vi "Periodic Tasks.vi"(8 "error in":errorcluster) -> ()   [LabVIEW 2013]
doc: "This VI runs in parallel to other tasks. It can contain as many user-defined periodic loops as you need. These can carry out PID or other sorts of timed response."
uses:
  <vilib>/Rock Robotics/SystemInterfaces/Utilities/FPGA_UtilitiesLED Source.ctl
  <vilib>/Rock Robotics/SystemInterfaces/Utilities/FPGA_UtilitiesLED State.ctl
  Robot Global Data.vi
panel:
  out "RDistance":dbl
  out "LDistance":dbl
  out "Distance":dbl
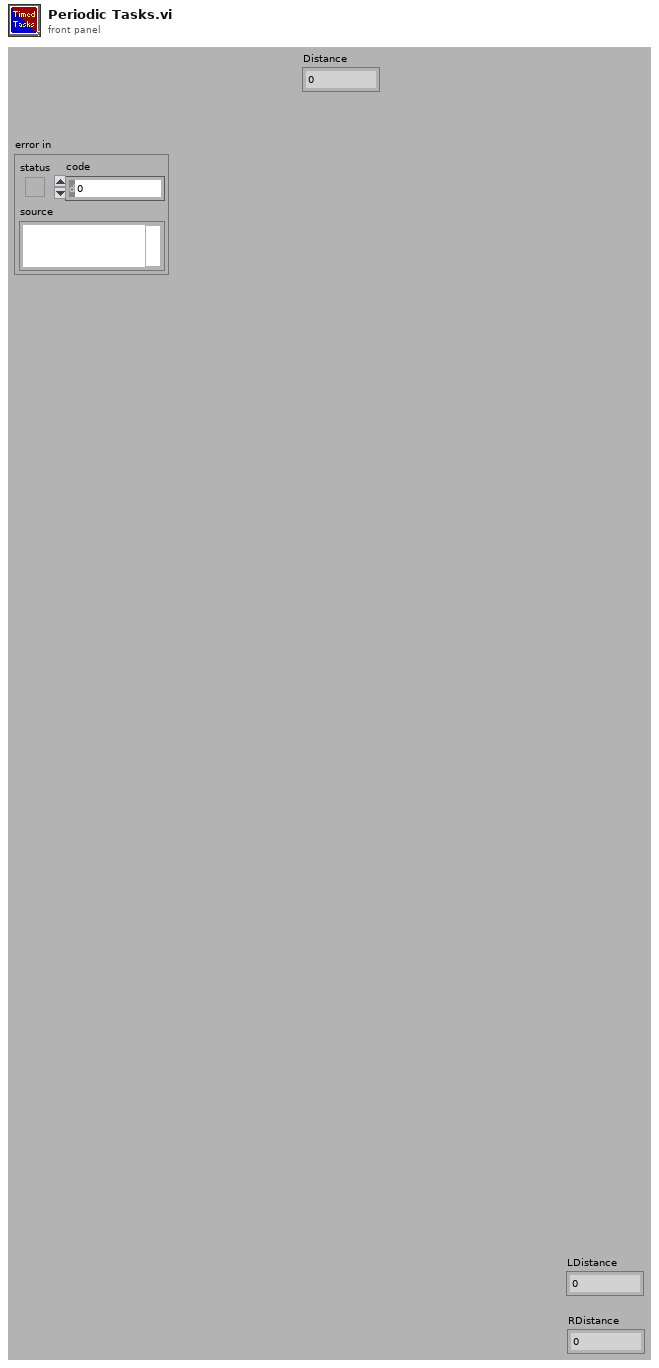
[diagram p1: front panel]
types:
  T1 = typedef "WPI_AnalogChannelDevRef.ctl" = cluster{"DevStatus":errorcluster, "Analog Module":T2, "Analog Channel":T3}
  T2 = typedef "FPGA_TypedefAnalogModule.ctl" = enum16{"Analog Module 1", "Analog Module 2"}
  T3 = typedef "FPGA_AIChannel.ctl" = enum8{"AI 1", "AI 2", "AI 3", "AI 4", "AI 5", "AI 6", "AI 7", "AI 8", "Invalid"}
  T4 = typedef "WPI_DigitalInputDevRef.ctl" = cluster{"DevStatus":errorcluster, "DIO Channel":T5, "Digital Module":T6}
  T5 = typedef "FPGA_DIOChannel.ctl" = enum8{"DIO 1", "DIO 2", "DIO 3", "DIO 4", "DIO 5", "DIO 6", "DIO 7", "DIO 8", "DIO 9", "DIO 10", "DIO 11", "DIO 12", "DIO 13", "DIO 14", "Invalid"}
  T6 = typedef "FPGA_TypedefDigitalModule.ctl" = enum16{"Digital Module 1", "Digital Module 2"}
  T7 = typedef "WPI_EncoderDevRef.ctl" = cluster{"DevStatus":errorcluster, "EncoderIndex":T8, "CounterIndex":T9, "DistancePerCount":dbl, "Decoding Type":T10}
  T8 = typedef "FPGA_EncoderIdx.ctl" = enum8{"Enc 0", "Enc 1", "Enc 2", "Enc 3", "Invalid"}
  T9 = typedef "FPGA_CounterCtrSystemIndex.ctl" = enum8{"Ctr 0", "Ctr 1", "Ctr 2", "Ctr 3", "Ctr 4", "Ctr 5", "Ctr 6", "Ctr 7", "Invalid"}
  T10 = typedef "WPI_EncoderType.ctl" = enum16{"1x", "2x", "4x"}
  T11 = cluster{"Winch Desired Location":dbl, "Winch Desired Location 2":dbl, "Winch Desired Location 3":dbl}
  T12 = typedef "FPGA_UtilitiesLED State.ctl" = enum16{"Off", "On", "Toggle"}
  T13 = typedef "FPGA_UtilitiesLED Source.ctl" = enum16{"User LED", "FPGA LED"}
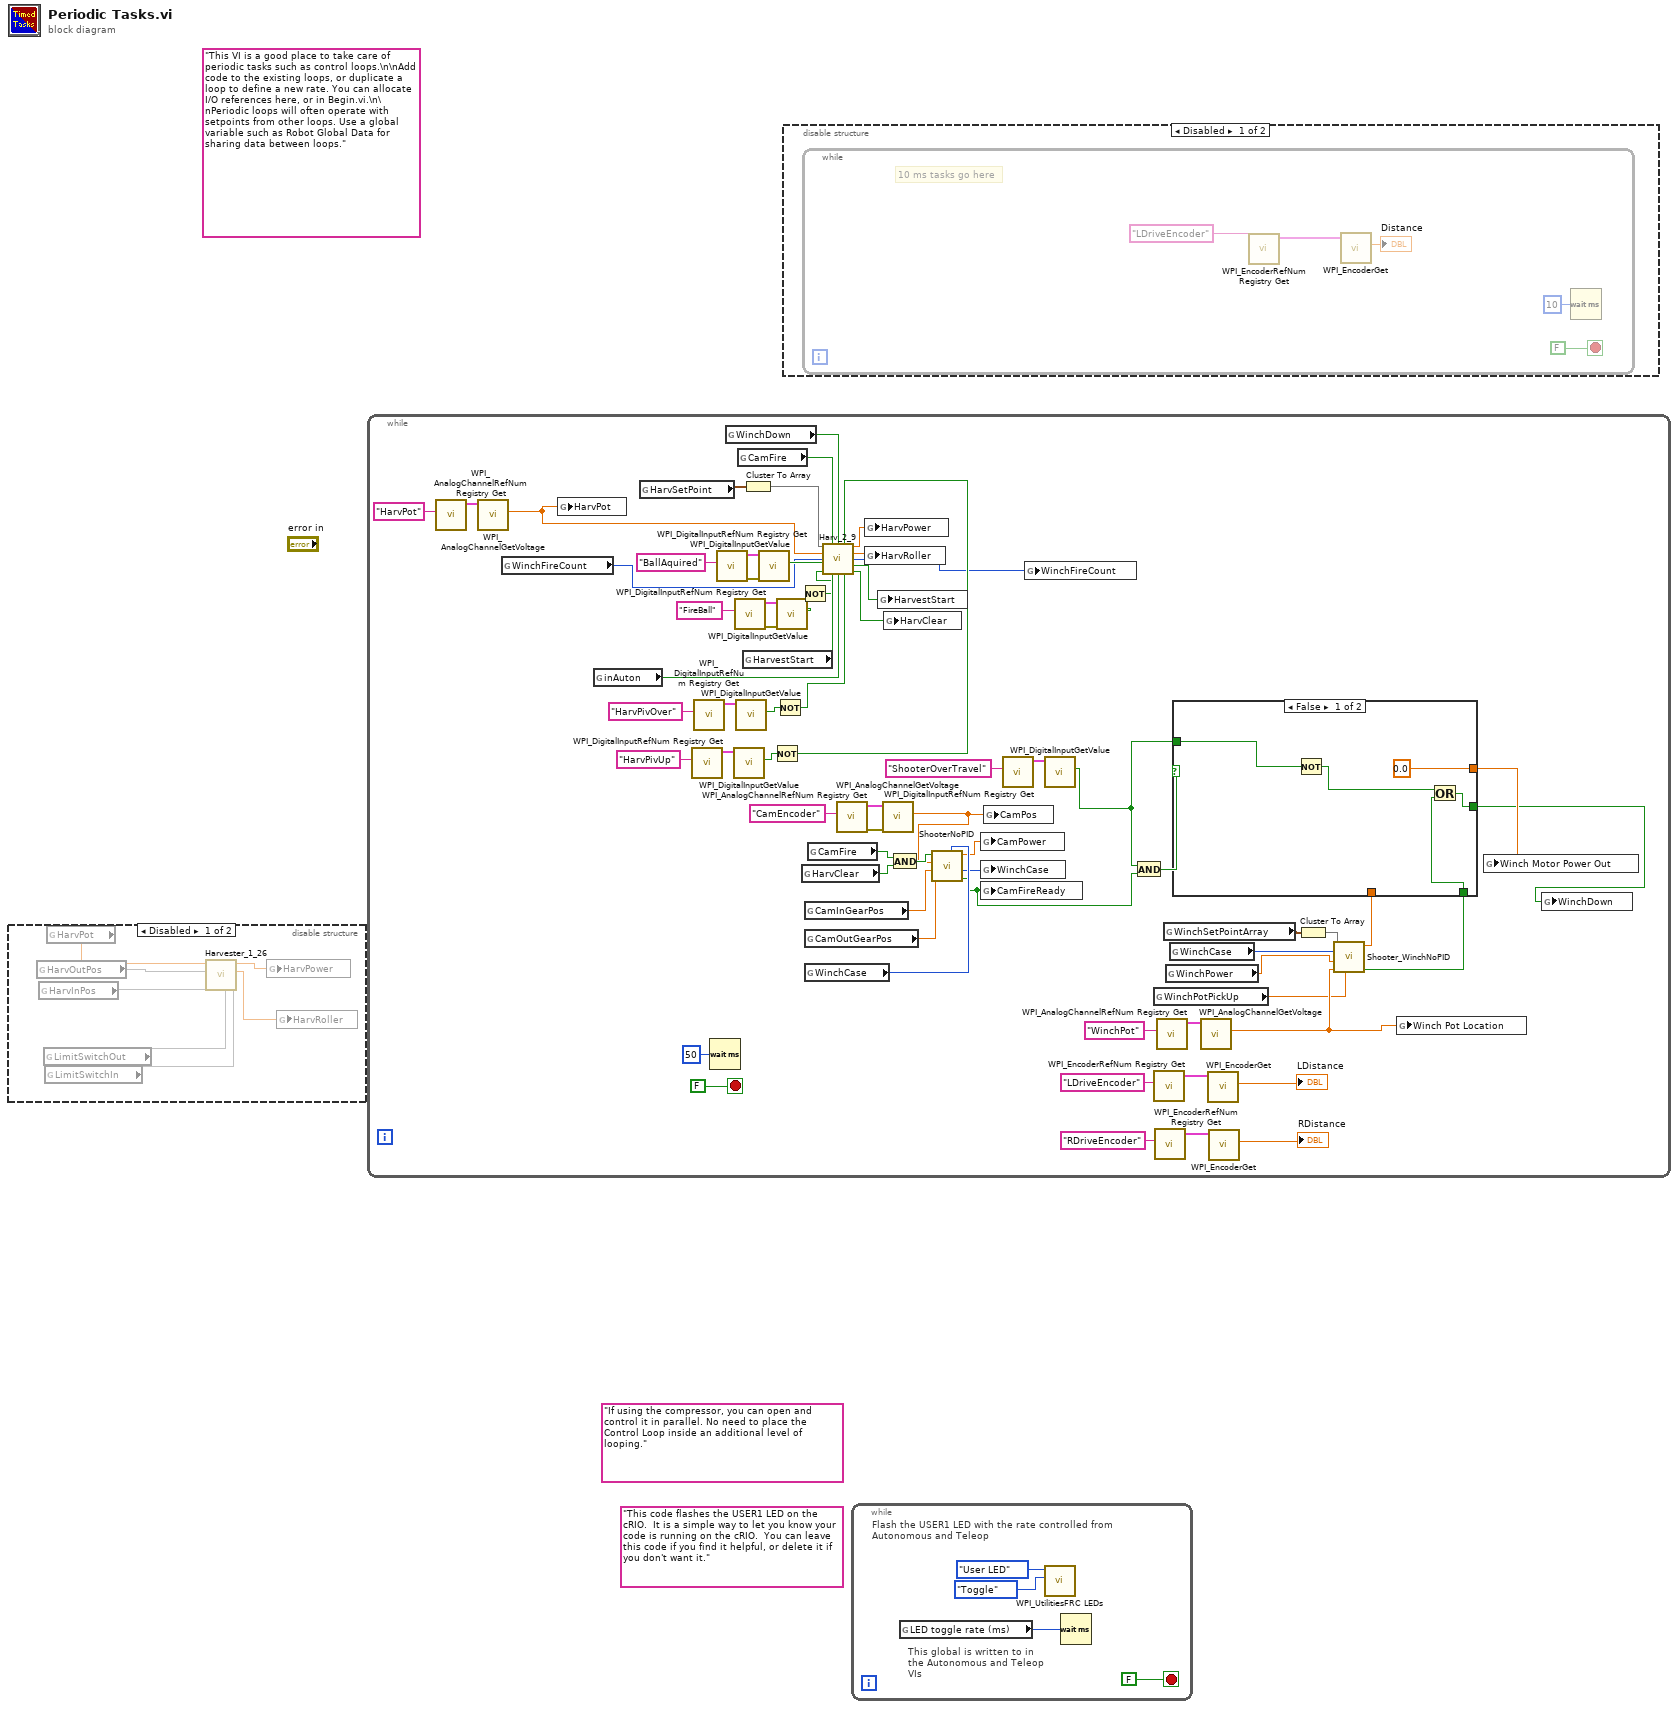
[diagram p0: block diagram]
diagram:
  (unwired) "If using the compressor, you can open and control it in parallel. No need to place the Control Loop inside an additional level of looping."
  (unwired) "This code flashes the USER1 LED on the cRIO.  It is a simple way to let you know your code is running on the cRIO.  You can leave this code if you find it helpful, or delete it if you don't want it."
  (unwired) "This VI is a good place to take care of periodic tasks such as control loops.\n\nAdd code to the existing loops, or duplicate a loop to define a new rate. You can allocate I/O references here, or in Begin.vi.\n\nPeriodic loops will often operate with setpoints from other loops. Use a global variable such as Robot Global Data for sharing data between loops."
  n1 = disable-structure shown="Disabled" {
    frame Disabled {
      n2 = global read "Robot Global Data.vi" "HarvOutPos"() -> (w6)
      n3 = global read "Robot Global Data.vi" "HarvInPos"() -> (w5)
      n4 = global read "Robot Global Data.vi" "LimitSwitchOut"() -> (w4)
      n5 = global read "Robot Global Data.vi" "LimitSwitchIn"() -> (w3)
      n6 = global read "Robot Global Data.vi" "HarvPot"() -> (w7:dbl)
      n7 = call "Harvester_1_26.vi"("LimitSwitchIn"=w3, "LimitSwitchOut"=w4, "HarvInPos"=w5, "HarvOutPos"=w6, "HarvPot"=w7) -> ("HarvRoller"=w2:dbl, "HarvPower"=w1:dbl)  [unwired: 5 in]
      n8 = global write "Robot Global Data.vi" "HarvPower"(w1) -> ()
      n9 = global write "Robot Global Data.vi" "HarvRoller"(w2) -> ()
    }
    frame Enabled {
    }
  }
  n10 = while {
    stop <- FALSE stop-if-true
    n11 = call <vilib>:"WPI_AnalogChannelRefNum Registry Get.vi"("refnum name"="HarvPot") -> ("AIDeviceRef"=w48:T1)  [unwired: 9 in, 1 out]
    n12 = call <vilib>:"WPI_AnalogChannelGetVoltage.vi"("AIDeviceRef"=w48) -> ("Voltage"=w20:dbl)  [unwired: 8 in, 2 out]
    n13 = global read "Robot Global Data.vi" "WinchFireCount"() -> (w9:i32)
    n14 = global write "Robot Global Data.vi" "HarvPot"(w20) -> ()
    n15 = global read "Robot Global Data.vi" "inAuton"() -> (w11:bool)
    n16 = global read "Robot Global Data.vi" "HarvSetPoint"() -> (w37:cluster{"Out":dbl, "In":dbl, "Clear":dbl})
    n17 = call <vilib>:"WPI_DigitalInputRefNum Registry Get.vi"("refnum name"="HarvPivUp") -> ("DigitalInputDevRef"=w57:T4)  [unwired: 9 in, 1 out]
    n18 = call <vilib>:"WPI_DigitalInputRefNum Registry Get.vi"("refnum name"="HarvPivOver") -> ("DigitalInputDevRef"=w66:T4)  [unwired: 9 in, 1 out]
    n19 = Wait (ms)(milliseconds to wait=u32 50) -> ()  [unwired: 1 out]
    n20 = call <vilib>:"WPI_DigitalInputRefNum Registry Get.vi"("refnum name"="BallAquired") -> ("error out"=w53:errorcluster, "DigitalInputDevRef"=w52:T4)  [unwired: 9 in]
    n21 = global read "Robot Global Data.vi" "WinchDown"() -> (w30:bool)
    n22 = call <vilib>:"WPI_DigitalInputGetValue.vi"("DigitalInputDevRef"=w57) -> ("Value"=w33:bool)  [unwired: 8 in, 2 out]
    n23 = call <vilib>:"WPI_DigitalInputRefNum Registry Get.vi"("refnum name"="FireBall") -> ("error out"=w44:errorcluster, "DigitalInputDevRef"=w45:T4)  [unwired: 9 in]
    n24 = call <vilib>:"WPI_DigitalInputGetValue.vi"("DigitalInputDevRef"=w66) -> ("Value"=w35:bool)  [unwired: 8 in, 2 out]
    n25 = global read "Robot Global Data.vi" "CamFire"() -> (w43:bool)
    n26 = Cluster To Array(cluster=w37) -> (array=w36:dbl[])
    n27 = global read "Robot Global Data.vi" "HarvestStart"() -> (w42:bool)
    n28 = call <vilib>:"WPI_DigitalInputGetValue.vi"("error in (no error)"=w53, "DigitalInputDevRef"=w52) -> ("Value"=w39:bool)  [unwired: 7 in, 2 out]
    n29 = Not(x=w33) -> (.not. x?=w32:bool)
    n30 = Not(x=w35) -> (.not. x?=w34:bool)
    n31 = call <vilib>:"WPI_DigitalInputGetValue.vi"("error in (no error)"=w44, "DigitalInputDevRef"=w45) -> ("Value"=w41:bool)  [unwired: 7 in, 2 out]
    n32 = Not(x=w41) -> (.not. x?=w38:bool)
    n33 = global read "Robot Global Data.vi" "HarvClear"() -> (w60:bool)
    n34 = global read "Robot Global Data.vi" "CamInGearPos"() -> (w16:dbl)
    n35 = global read "Robot Global Data.vi" "CamOutGearPos"() -> (w15:dbl)
    n36 = global read "Robot Global Data.vi" "WinchCase"() -> (w18:i32)
    n37 = global read "Robot Global Data.vi" "CamFire"() -> (w59:bool)
    n38 = call "Harv_2_9.vi"("HarvSetpoints"=w36, "Fire"=w43, "WinchDown"=w30, "HarvPivUP"=w32, "HarvPot"=w20, "Count"=w9, "BallAcquired"=w39, "FireBallSen"=w38, "Harvest"=w42, "inAuton?"=w11, "HarvPivPickupLim"=w34) -> ("HarvPower"=w50:dbl, "HarvRoller"=w49:dbl, "CountOut"=w8:i32, "HarvStart"=w31:bool, "HarvCleared"=w40:bool)
    n39 = call <vilib>:"WPI_AnalogChannelRefNum Registry Get.vi"("refnum name"="CamEncoder") -> ("error out"=w62:errorcluster, "AIDeviceRef"=w61:T1)  [unwired: 9 in]
    n40 = global write "Robot Global Data.vi" "HarvPower"(w50) -> ()
    n41 = global write "Robot Global Data.vi" "HarvRoller"(w49) -> ()
    n42 = global write "Robot Global Data.vi" "HarvestStart"(w31) -> ()
    n43 = call <vilib>:"WPI_AnalogChannelGetVoltage.vi"("error in (no error)"=w62, "AIDeviceRef"=w61) -> ("Voltage"=w17:dbl)  [unwired: 7 in, 2 out]
    n44 = global write "Robot Global Data.vi" "HarvClear"(w40) -> ()
    n45 = And(x=w59, y=w60) -> (x .and. y?=w19:bool)
    n46 = call "ShooterNoPID.vi"("WinchCaseIn"=w18, "InGearPosLow"=w15, "InGearPosHigh"=w16, "Pot"=w17, "Fire"=w19) -> ("There?"=w12:bool, "WinchCase"=w13:i32, "Power"=w14:dbl)  [unwired: 4 in]
    n47 = global write "Robot Global Data.vi" "CamPower"(w14) -> ()
    n48 = global write "Robot Global Data.vi" "WinchCase"(w13) -> ()
    n49 = global write "Robot Global Data.vi" "CamFireReady"(w12) -> ()
    n50 = global write "Robot Global Data.vi" "CamPos"(w17) -> ()
    n51 = call <vilib>:"WPI_DigitalInputRefNum Registry Get.vi"("refnum name"="ShooterOverTravel") -> ("DigitalInputDevRef"=w56:T4)  [unwired: 9 in, 1 out]
    n52 = global write "Robot Global Data.vi" "WinchFireCount"(w8) -> ()
    n53 = call <vilib>:"WPI_DigitalInputGetValue.vi"("DigitalInputDevRef"=w56) -> ("Value"=w29:bool)  [unwired: 8 in, 2 out]
    n54 = And(x=w29, y=w12) -> (x .and. y?=w54:bool)
    n55 = global read "Robot Global Data.vi" "WinchPotPickUp"() -> (w10:dbl)
    n56 = call <vilib>:"WPI_EncoderRefNum Registry Get.vi"("refnum name"="LDriveEncoder") -> ("EncoderDevRef"=w71:T7)  [unwired: 9 in, 1 out]
    n57 = call <vilib>:"WPI_EncoderRefNum Registry Get.vi"("refnum name"="RDriveEncoder") -> ("EncoderDevRef"=w68:T7)  [unwired: 9 in, 1 out]
    n58 = call <vilib>:"WPI_AnalogChannelRefNum Registry Get.vi"("refnum name"="WinchPot") -> ("AIDeviceRef"=w73:T1)  [unwired: 9 in, 1 out]
    n59 = global read "Robot Global Data.vi" "WinchSetPointArray"() -> (w26:T11)
    n60 = global read "Robot Global Data.vi" "WinchPower"() -> (w28:dbl)
    n61 = global read "Robot Global Data.vi" "WinchCase"() -> (w25:i32)
    n62 = call <vilib>:"WPI_AnalogChannelGetVoltage.vi"("AIDeviceRef"=w73) -> ("Voltage"=w24:dbl)  [unwired: 8 in, 2 out]
    n63 = call <vilib>:"WPI_EncoderGet.vi"("EncoderDevRef"=w71) -> ("Distance"=→"LDistance":dbl)  [unwired: 5 in, 5 out]
    n64 = call <vilib>:"WPI_EncoderGet.vi"("EncoderDevRef"=w68) -> ("Distance"=→"RDistance":dbl)  [unwired: 5 in, 5 out]
    n65 = Cluster To Array(cluster=w26) -> (array=w27:dbl[])
    n66 = call "Shooter_WinchNoPID.vi"("PickStartPos"=w10, "Winch Pot Location"=w24, "WinchPower"=w28, "selectedCase"=w25, "SetPointArray"=w27) -> ("isThere?"=w22:bool, "Winch Motor Power Out"=w21:dbl)  [unwired: 5 in]
    n67 = case shown="False" w54 {
      tunnel: [0.0 ("Winch Motor Power Out") w82] -> w64
      tunnel: [w80 w83] -> w23
      tunnel: w29 -> [w79 _]
      tunnel: w22 -> [w77 w83]
      tunnel: w21 -> [_ w82]
      frame False {
        n68 = Not(x=w79) -> (.not. x?=w78:bool)
        n69 = Or(x=w78, y=w77) -> (x .or. y?=w80:bool)
      }
      frame True {
      }
    }
    n70 = global write "Robot Global Data.vi" "Winch Pot Location"(w24) -> ()
    n71 = global write "Robot Global Data.vi" "Winch Motor Power Out"(w64) -> ()
    n72 = global write "Robot Global Data.vi" "WinchDown"(w23) -> ()
  }
  n73 = disable-structure shown="Disabled" {
    frame Disabled {
      n74 = while {
        stop <- FALSE stop-if-true
        # "10 ms tasks go here"
        n75 = call <vilib>:"WPI_EncoderRefNum Registry Get.vi"("refnum name"="LDriveEncoder") -> ("EncoderDevRef"=w84:T7)  [unwired: 9 in, 1 out]
        n76 = call <vilib>:"WPI_EncoderGet.vi"("EncoderDevRef"=w84) -> ("Distance"=→"Distance":dbl)  [unwired: 5 in, 5 out]
        n77 = Wait (ms)(milliseconds to wait=u32 10) -> ()  [unwired: 1 out]
      }
    }
    frame Enabled {
    }
  }
  n78 = while {
    stop <- FALSE stop-if-true
    # "This global is written to in the Autonomous and Teleop VIs"
    # "Flash the USER1 LED with the rate controlled from Autonomous and Teleop"
    n79 = global read "Robot Global Data.vi" "LED toggle rate (ms)"() -> (w89:u32)
    n80 = call <vilib>:"WPI_UtilitiesFRC LEDs.vi"("State"=FPGA_UtilitiesLED_State."Toggle", "LED Type"=FPGA_UtilitiesLED_Source."User LED") -> ()  [unwired: 1 in, 9 out]
    n81 = Wait (ms)(milliseconds to wait=w89) -> ()  [unwired: 1 out]
  }
